vi "elevateur.vi"(1 "Elevateur":dbl, 2 "Crochet":bool) -> ()   [LabVIEW 2019]
uses:
  <vilib>/Rock Robotics/WPI/ThirdParty/Phoenix-LabVIEW/Motor Controller/Controls/CTRE_Phoenix_MotorControl_ControlMode.ctl
  <vilib>/Rock Robotics/WPI/Solenoid/WPI_SolenoidValue.ctl
  <vilib>/Rock Robotics/WPI/ThirdParty/Phoenix-LabVIEW/Motor Controller/Get/CTRE_Phoenix_MotorController_GetQuadratureData.vi
  <vilib>/Rock Robotics/Network Tables/NT Write Number.vi
  <vilib>/Rock Robotics/WPI/Solenoid/WPI_SolenoidSetEnum.vi
  Robot Global Data.vi
  <vilib>/Rock Robotics/Network Tables/NT Write Boolean.vi
panel:
  in  "Bypass":bool
  out "Quadrature Position":i32
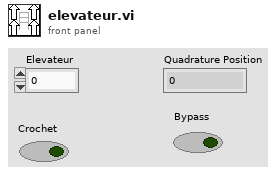
[diagram p1: front panel]
types:
  T1 = typedef "WPI_SolenoidValue.ctl" = enum16{"Off", "On", "Forward", "Reverse"}
  T2 = typedef "CTRE_Phoenix_MotorControl_ControlMode.ctl" = u16
  T3 = typedef "WPI_SwitchDevRef.ctl" = cluster{"DevStatus":errorcluster, "DIO Channel":T4, "CntIndex":T5, "Normally Closed":bool}
  T4 = typedef "FPGA_DIOChannel.ctl" = enum8{"DIO 0", "DIO 1", "DIO 2", "DIO 3", "DIO 4", "DIO 5", "DIO 6", "DIO 7", "DIO 8", "DIO 9", "DIO MXP 0", "DIO MXP 1", "DIO MXP 2", "DIO MXP 3", "DIO MXP 4", "DIO MXP 5", "DIO MXP 6", "DIO MXP 7", "DIO MXP 8", "DIO MXP 9", "DIO MXP 10", "DIO MXP 11", "DIO MXP 12", "DIO MXP 13", "DIO MXP 14", "DIO MXP 15", "SPI Port CS1", "SPI Port CS2", "SPI Port CS3", "SPI Port MISO", "SPI Port MOSI", "Invalid"}
  T5 = typedef "FPGA_CounterCtrSystemIndex.ctl" = enum8{"Ctr 0", "Ctr 1", "Ctr 2", "Ctr 3", "Ctr 4", "Ctr 5", "Ctr 6", "Ctr 7", "Invalid"}
  T6 = typedef "WPI_MotorControlDeviceRef.ctl" = cluster{"DeviceStatus":errorcluster, "Type":T7, "PWM":cluster{"PWM Channel":T8, "DeadBand":T9}, "CAN":cluster{"Device Number":u8, "SetOutput VI Ref":variant, "GetOutput VI Ref":variant, "Enable VI Ref":variant, "Disable VI Ref":variant, "Data":variant}, "Invert":bool, "DIO PWM":cluster{"PWM \"Enable\" Channel":T8, "DIOChannel":T4, "PWM Rate":dbl}}
  T7 = typedef "WPI_MotorControlType.ctl" = enum16{"PWM", "CAN", "DIO PWM"}
  T8 = typedef "FPGA_DIOPWMChannel.ctl" = enum8{"PWM 0", "PWM 1", "PWM 2", "PWM 3", "PWM 4", "PWM 5", "PWM 6", "PWM 7", "PWM 8", "PWM 9", "PWM MXP 0", "PWM MXP 1", "PWM MXP 2", "PWM MXP 3", "PWM MXP 4", "PWM MXP 5", "PWM MXP 6", "PWM MXP 7", "PWM MXP 8", "PWM MXP 9", "Invalid"}
  T9 = typedef "WPI_PWMDeadband.ctl" = cluster{"Name":string, "maxPositivePwm":i32, "minPositivePwm":i32, "centerPwm":i32, "maxNegativePwm":i32, "minNegativePwm":i32, "angularRange":u16}
  T10 = typedef "WPI_SolenoidDevRef.ctl" = cluster{"DevStatus":errorcluster, "Pneumatics Control Module":u8, "Forward Solenoid Channel":T11, "Reverse Solenoid Channel":T11}
  T11 = typedef "WPI_SolenoidChannel.ctl" = enum8{"Solenoid 0", "Solenoid 1", "Solenoid 2", "Solenoid 3", "Solenoid 4", "Solenoid 5", "Solenoid 6", "Solenoid 7", "Invalid"}
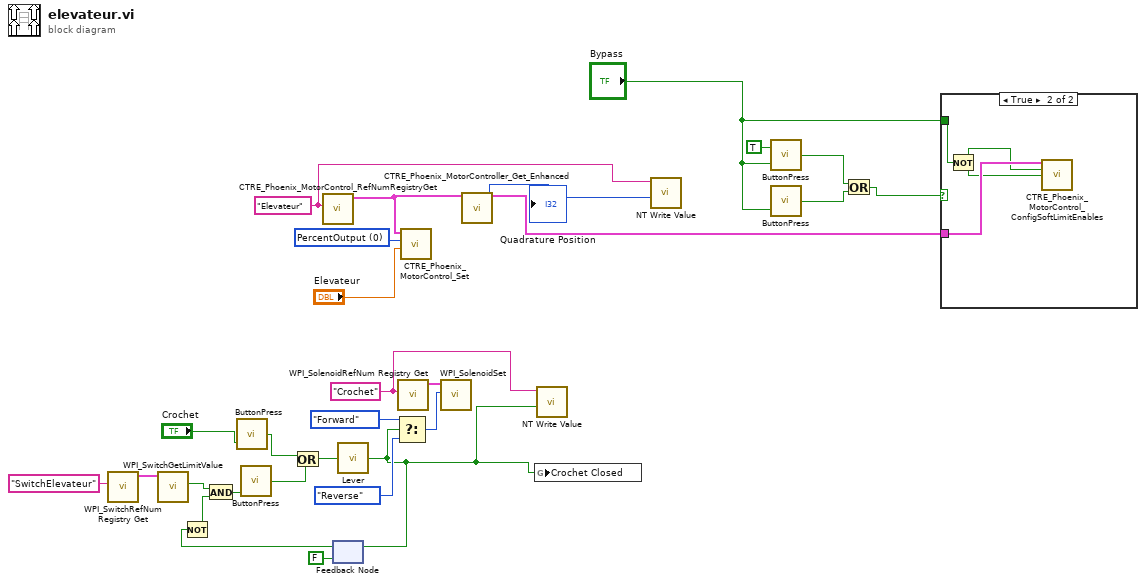
[diagram p0: block diagram]
diagram:
  w19 = "Crochet" ("refnum name")
  w28 = T2 0 items=["PercentOutput"=0, "Position"=1, "Velocity"=2, "Current"=3, "Follower"=5, "MotionProfile"=6, "MotionMagic"=7, "MotionProfileArc"=10, "Disabled"=15] ("Control Mode")
  w26 = "Elevateur" ("refnum name")
  n1 = call <vilib>:"WPI_SwitchRefNum Registry Get.vi"("refnum name"="SwitchElevateur") -> ("SwitchDevRef"=w12:T3)  [unwired: 9 in, 1 out]
  n2 = call <vilib>:"WPI_SwitchGetLimitValue.vi"("SwitchDevRef"=w12) -> ("Switch Pressed"=w6:bool)  [unwired: 8 in, 2 out]
  n3 = call "ButtonPress.vi"("Input"="Crochet") -> ("Output"=w9:bool)  [unwired: 1 in]
  n4 = call <vilib>:"CTRE_Phoenix_MotorControl_RefNumRegistryGet.vi"("refnum name"=w26) -> ("PhoenixMotorControlDevRef"=w27:T6)  [unwired: 9 in, 1 out]
  n5 = feedback #1(FALSE ("Output")) -> (w2:bool)
  n6 = Not(x=w2) -> (.not. x?=w4:bool)
  n7 = And(x=w6, y=w4) -> (x .and. y?=w5:bool)
  n8 = call "ButtonPress.vi"("Input"=w5) -> ("Output"=w8:bool)  [unwired: 1 in]
  n9 = Or(x=w9, y=w8) -> (x .or. y?=w7:bool)
  n10 = call "Lever.vi"("Input"=w7) -> ("Output"=w3:bool)
  n11 = feedback-in #1(w3) -> ()
  n12 = Select(t=WPI_SolenoidValue."Forward" ("Value"), s=w3, f=WPI_SolenoidValue."Reverse" ("Value")) -> (s? t:f=w21:T1)
  n13 = call <vilib>:"WPI_SolenoidRefNum Registry Get.vi"("refnum name"=w19) -> ("SolenoidDevRef"=w23:T10)  [unwired: 9 in, 1 out]
  n14 = call <vilib>:"CTRE_Phoenix_MotorControl_Set.vi"("Output"="Elevateur", "Control Mode"=w28, "PhoenixMotorControlDevRef"=w27) -> ()  [unwired: 7 in, 2 out]
  n15 = call-poly <vilib>:"WPI_SolenoidSet.vi"("Value"=w21, "SolenoidDevRef"=w23) -> ()  [unwired: 8 in, 2 out]
  n16 = call-poly <vilib>:"CTRE_Phoenix_MotorController_Get_Enhanced.vi"("PhoenixMotorControlDevRef"=w27) -> ("PhoenixMotorControlDevRef"=w16:T6, "Quadrature Position"=w25:i32)  [unwired: 11 in, 2 out]
  "Quadrature Position" <- w25
  n17 = global write "Robot Global Data.vi" "Crochet Closed"(w3) -> ()
  n18 = call-poly <vilib>:"NT Write Value.vi"("Boolean"=w3, "Name"=w19) -> ()  [unwired: 9 in, 1 out]
  n19 = call-poly <vilib>:"NT Write Value.vi"("Numeric"=w25, "Name"=w26) -> ()  [unwired: 9 in, 1 out]
  n20 = call "ButtonPress.vi"("Input"="Bypass", "Falling Edge?"=TRUE) -> ("Output"=w18:bool)
  n21 = call "ButtonPress.vi"("Input"="Bypass") -> ("Output"=w17:bool)  [unwired: 1 in]
  n22 = Or(x=w18, y=w17) -> (x .or. y?=w14:bool)
  n23 = case shown="True" w14 {
    tunnel: w16 -> [_ w31]
    tunnel: "Bypass" -> [_ w29]
    frame False {
    }
    frame True {
      n24 = Not(x=w29) -> (.not. x?=w30:bool)
      n25 = call <vilib>:"CTRE_Phoenix_MotorControl_ConfigSoftLimitEnables.vi"("PhoenixMotorControlDevRef"=w31, "Forward Soft Limit Enable"=w30, "Reverse Soft Limit Enable"=w30) -> ()  [unwired: 11 in, 2 out]
    }
  }
